vi "ToJson.vi"(8 "error in (no error)":errorcluster, 11 "Flags in":refnum<class "Flags.lvclass">) -> (0 "error out":errorcluster, 2 "String":string, 3 "Flags out":refnum<class "Flags.lvclass">)   [LabVIEW 2015, in "Flags.lvclass"]
uses:
  Flags.lvclass
  JasonCluster.ctl
  Flags.lvclass/Flags.ctl
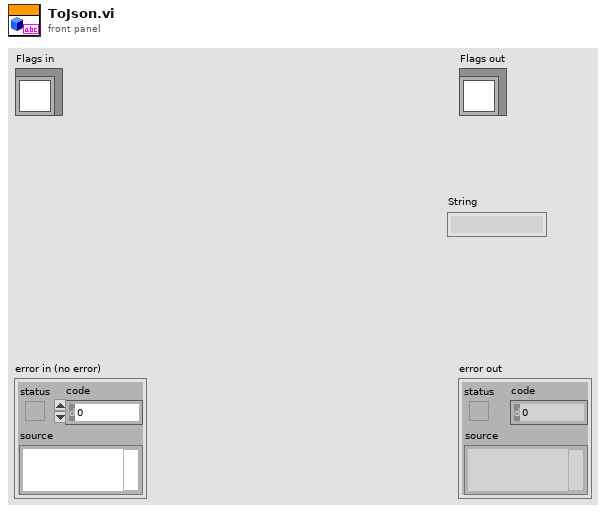
[diagram p1: front panel]
types:
  T1 = typedef "Flags.lvclass/JasonCluster.ctl" = cluster{"State":bool[], "Color":i32[]}
  T2 = typedef "Flags.lvclass/ColorEnum.ctl" = enum8{"Red", "Blue", "Green", "Yellow"}
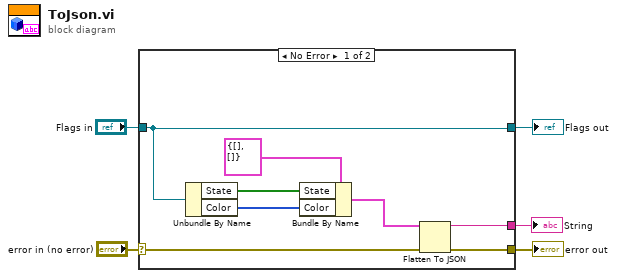
[diagram p0: block diagram]
diagram:
  n1 = case shown="No Error" "error in (no error)" {
    selector: "error in (no error)" -> [w8 w15]
    tunnel: [w7 w15] -> w4
    tunnel: [w13 w14] -> w2
    tunnel: "Flags in" -> [w13 w14]
    tunnel: [w6 _] -> w1
    frame No Error {
      n2 = Unbundle By Name(w13) -> ("State"=w11:bool[], "Color"=w10:T2[])
      n3 = Bundle By Name(cluster=T1 {"State"=[], "Color"=[]} ("Cluster of class private data"), "State"=w11, "Color"=w10) -> (w9:T1)
      n4 = Flatten To JSON(anything=w9, error in (no error)=w8) -> (JSON string=w6:string, 11:w7:errorcluster)  [unwired: 1 in]
    }
    frame Error {
    }
  }
  "error out" <- w4
  "Flags out" <- w2
  "String" <- w1
